vi "runtime execution.vi"() -> (0 "error out":errorcluster, 2 "success?":bool)   [LabVIEW 2013, in "shared memory tests.lvlib"]
uses:
  shared memory tests.lvlib
  module/execution/Shared Memory Runtime.lvclass
  <vilib>/NI/Tag Bus Module Framework/channel/channel classification.ctl
  module/configuration/shared memory configuration.lvclass
  module/execution/Read processing parameters.vi
  module/execution/Read processing results.vi
  <vilib>/National Instruments/Shared Memory Library for Linux RT/Classes/Shared Memory/Shared Memory.lvclass
  <vilib>/NI/Tag Bus Module Framework/channel/TBM channel.lvclass
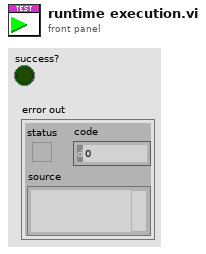
[diagram p1: front panel]
types:
  T1 = typedef "TBM channel.lvclass/channel classification.ctl" = enum16{"input data", "output data", "processing parameter", "processing result"}
  T2 = typedef "TBM channel.lvclass/data tables.ctl" = cluster{"input data":T3, "processing parameter":T3, "processing result":T3, "output data":T3}
  T3 = typedef "tag bus.lvlib/dictionary table pair.ctl" = cluster{"data dictionary":refnum<class "data dictionary.lvclass">, "data table":T4}
  T4 = typedef "tag bus.lvlib/data table.lvlib/data table.ctl" = cluster{"Double":dbl[], "Single":sgl[], "I64":i64[], "I32":i32[], "I16":i16[], "I8":i8[], "U64":u64[], "U32":u32[], "U16":u16[], "U8":u8[], "Boolean":bool[], "String":string[], "Array of Double":cluster{"DBL Array":dbl[]}[], "Array of Single":cluster{"SGL Array":sgl[]}[], "Array of I64":cluster{"I64 Array":i64[]}[], "Array of I32":cluster{"I32 Array":i32[]}[], "Array of I16":cluster{"I16 Array":i16[]}[], "Array of I8":cluster{"I8 Array":i8[]}[], "Array of U64":cluster{"U64 Array":u64[]}[], "Array of U32":cluster{"U32 Array":u32[]}[], "Array of U16":cluster{"U16 Array":u16[]}[], "Array of U8":cluster{"U8 Array":u8[]}[], "Array of Boolean":cluster{"Boolean Array":bool[]}[], "Array of String":cluster{"String Array":string[]}[]}
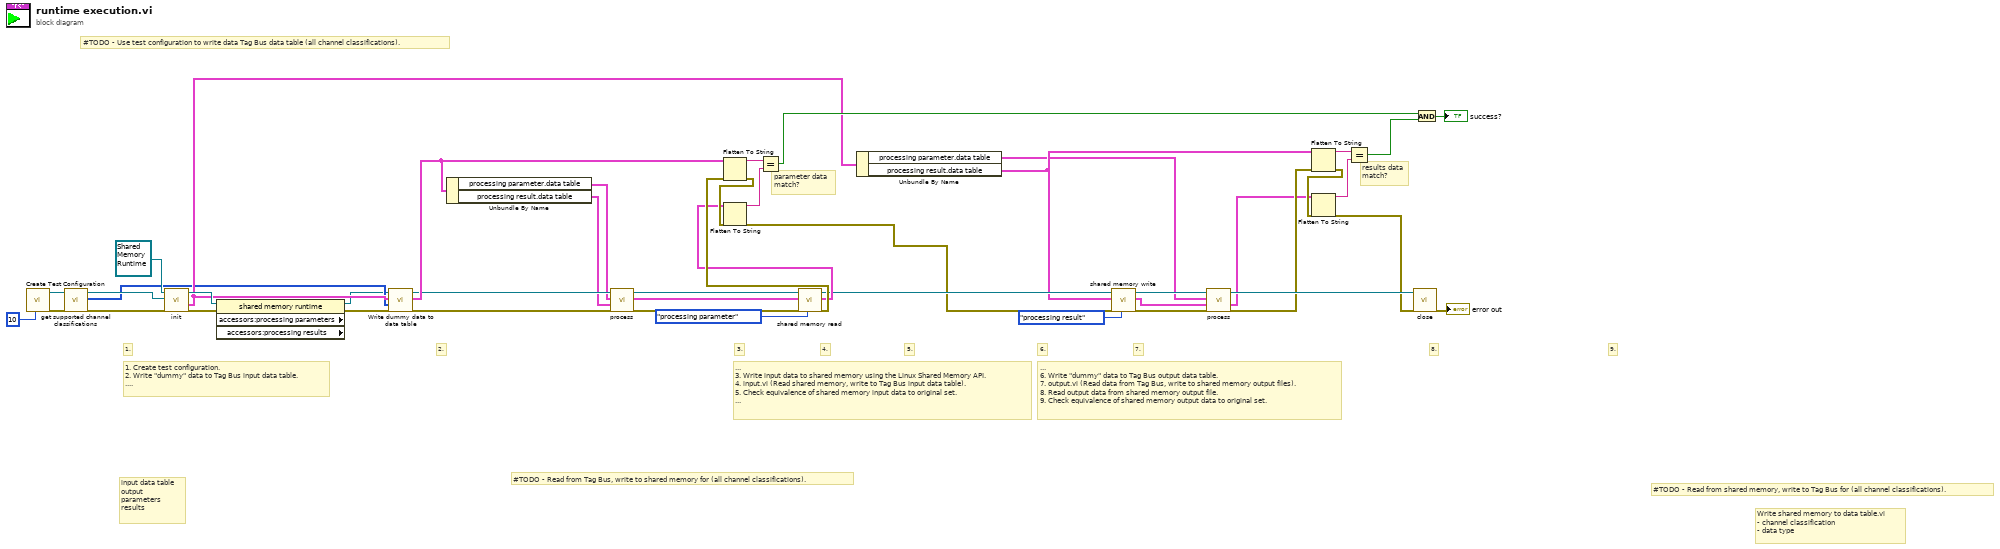
[diagram p0: block diagram]
diagram:
  # "results data\nmatch?"
  # "parameter data\nmatch?"
  # "Write shared memory to data table.vi\n- channel classification\n- data type"
  # "#TODO - Read from shared memory, write to Tag Bus for (all channel classifications)."
  # "#TODO - Read from Tag Bus, write to shared memory for (all channel classifications)."
  # "input data table\noutput\nparameters\nresults"
  # "#TODO - Use test configuration to write data Tag Bus data table (all channel classifications)."
  # "...\n6. Write \"dummy\" data to Tag Bus output data table.\n7. output.vi (Read data from Tag Bus, write to shared memory output files).\n8. Read output data from shared memory output file.\n9. Check equivalence of shared memory output data to original set."
  # "...\n3. Write input data to shared memory using the Linux Shared Memory API.\n4. input.vi (Read shared memory, write to Tag Bus input data table).\n5. Check equivalence of shared memory input data to original set.\n..."
  # "9."
  # "6."
  # "8."
  # "5."
  # "7."
  # "4."
  # "3."
  # "2."
  # "1."
  # "1. Create test configuration.\n2. Write \"dummy\" data to Tag Bus input data table.\n...."
  n1 = call "Create Test Configuration.vi"("number of channels per data type (1)"=10) -> ("error out"=w37:errorcluster, "Module Configuration"=w35:refnum<class "shared memory configuration.lvclass">)  [unwired: 5 in, 4 out]
  n2 = call-dynamic "get supported channel classifications.vi"("error in"=w37, "module configuration in"=w35) -> ("error out"=w36:errorcluster, "supported classifications"=w32:T1[], "module configuration out"=w34:refnum<class "shared memory configuration.lvclass">)  [unwired: 7 in]
  n3 = call-dynamic "init.vi"("error in"=w36, "TBM module configuration in"=w34, "shared memory runtime in"=refnum<class "Shared Memory Runtime.lvclass"> refnum ("tag bus configurable plugin module")) -> ("error out"=w44:errorcluster, "data allocations"=w33:T2, "shared memory runtime out"=w43:refnum<class "Shared Memory Runtime.lvclass">)  [unwired: 5 in, 1 out]
  n4 = property class="shared memory runtime" props=["accessors:processing parameters", "accessors:processing results"](reference=w43, error in=w44) -> (reference out=w28:refnum<class "Shared Memory Runtime.lvclass">, error out=w31:errorcluster)  [unwired: 2 out]
  n5 = call "Write dummy data to data table.vi"("shared memory runtime"=w28, "data allocations"=w33, "supported classifications"=w32, "error in"=w31) -> ("shared memory runtime out"=w27:refnum<class "Shared Memory Runtime.lvclass">, "data allocations out"=w29:T2, "error out"=w30:errorcluster)  [unwired: 4 in]
  n6 = Unbundle By Name(w29) -> ("processing parameter.data table"=w21:T4, "processing result.data table"=w2:T4)
  n7 = call-dynamic "process.vi"("error in"=w30, "results data"=w2, "parameters data"=w21, "module in"=w27) -> ("error out"=w20:errorcluster, "parameter data out"=w12:T4, "module out"=w19:refnum<class "Shared Memory Runtime.lvclass">)  [unwired: 4 in, 1 out]
  n8 = call "shared memory read.vi"("channel classification"=channel_classification."processing parameter", "error in"=w20, "data table"=w12, "module in"=w19) -> ("error out"=w17:errorcluster, "data table out"=w16:T4, "module out"=w15:refnum<class "Shared Memory Runtime.lvclass">)  [unwired: 5 in]
  n9 = Flatten To String(anything=w29, error in (no error)=w17) -> (data string=w24:string, error out=w22:errorcluster)  [unwired: 2 in, 1 out]
  n10 = Flatten To String(anything=w16, error in (no error)=w22) -> (data string=w23:string, error out=w14:errorcluster)  [unwired: 2 in, 1 out]
  n11 = Equal?(x=w24, y=w23) -> (x = y?=w40:bool)
  n12 = Unbundle By Name(w33) -> ("processing parameter.data table"=w1:T4, "processing result.data table"=w4:T4)
  n13 = call "shared memory write.vi"("channel classification"=channel_classification."processing result", "error in"=w14, "data table"=w4, "module in"=w15) -> ("error out"=w10:errorcluster, "data table out"=w9:T4, "module out"=w11:refnum<class "Shared Memory Runtime.lvclass">)  [unwired: 5 in]
  n14 = call-dynamic "process.vi"("error in"=w10, "results data"=w9, "parameters data"=w1, "module in"=w11) -> ("error out"=w5:errorcluster, "results data out"=w3:T4, "module out"=w41:refnum<class "Shared Memory Runtime.lvclass">)  [unwired: 4 in, 1 out]
  n15 = Flatten To String(anything=w4, error in (no error)=w5) -> (data string=w6:string, error out=w8:errorcluster)  [unwired: 2 in, 1 out]
  n16 = Flatten To String(anything=w3, error in (no error)=w8) -> (data string=w7:string, error out=w25:errorcluster)  [unwired: 2 in, 1 out]
  n17 = Equal?(x=w6, y=w7) -> (x = y?=w26:bool)
  n18 = call-dynamic "close.vi"("error in"=w25, "shared memory runtime"=w41) -> ("error out"=→"error out":errorcluster)  [unwired: 9 in]
  n19 = And(x=w40, y=w26) -> (x .and. y?=→"success?":bool)
